vi "RSZVB Set TRM Combiner State.vi"(7 "Combiner State (Off)":bool, 8 "error in (no error)":errorcluster {"code" format="%.0x"}, 9 "Path (1)":i32=1, 10 "Channel (1)":i32=1, 11 "VISA resource name":refnum<visa-resource-name>) -> (0 "error out":errorcluster {"code" format="%.0x"}, 3 "VISA resource name out":refnum<visa-resource-name>)   [LabVIEW 2011]
doc: "This VI switches the internal combiner in-between RF signal paths 1 and 3 or 2 and 4 (source path).\n\nRemote-control command(s):\n[SENSe<Ch>:]TEUNit:COMBiner<Path>[:STATe]"
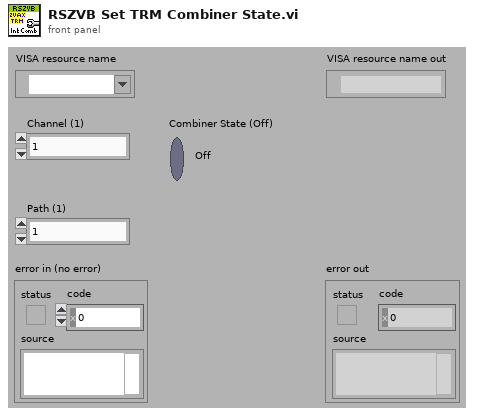
[diagram p1: front panel]
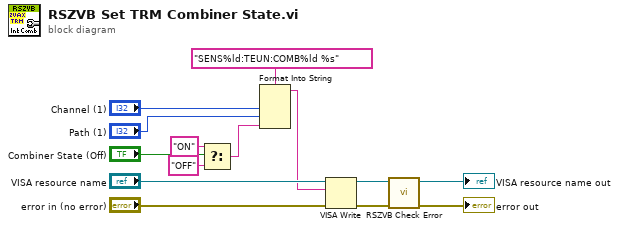
[diagram p0: block diagram]
diagram:
  n1 = Select(t="ON", s="Combiner State (Off)", f="OFF") -> (s? t:f=w5:string)
  n2 = Format Into String(format string="SENS%ld:TEUN:COMB%ld %s", "Channel (1)", "Path (1)", w5) -> (resulting string=w2:string)  [unwired: 2 in, 1 out]
  n3 = VISA Write(VISA resource name="VISA resource name", write buffer=w2, error in (no error)="error in (no error)") -> (VISA resource name out=w13:refnum<visa-resource-name>, error out=w14:errorcluster)  [unwired: 1 out]
  n4 = call "RSZVB Check Error.vi"("error in (no error)"=w14, "VISA session"=w13) -> ("error out"=→"error out":errorcluster, "dup VISA session"=→"VISA resource name out":refnum<visa-resource-name>)  [unwired: 8 in]
